vi "Read Logging Interval.vi"(8 "error in (no error)":errorcluster, 11 "Data Logger in":refnum<class "Data Logger.lvclass">) -> (0 "error out":errorcluster, 2 "Logging Interval":dbl=1.0 min=1.0 step=1.0 format="%<%H:%M:%S>t", 3 "Data Logger out":refnum<class "Data Logger.lvclass">)   [LabVIEW 2014, in "Data Logger.lvlib" / "Data Logger.lvclass"]
uses:
  Data Logger.lvclass
  Data Logger.lvclass/Data Logger.ctl
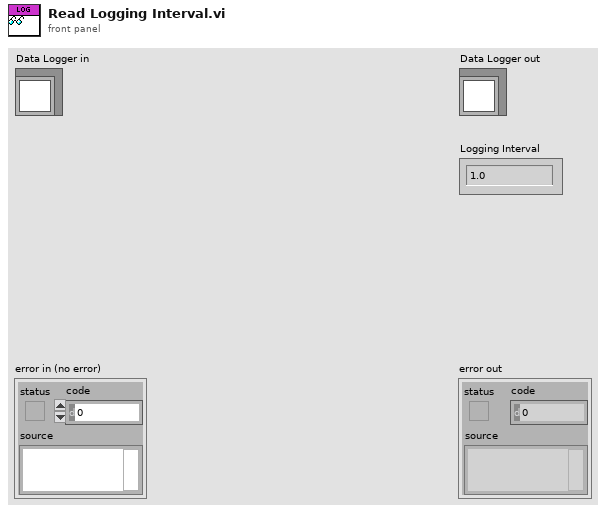
[diagram p1: front panel]
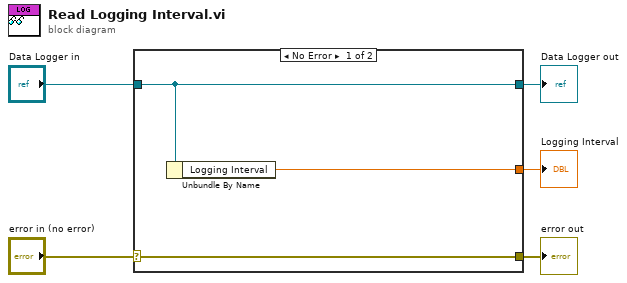
[diagram p0: block diagram]
diagram:
  n1 = case shown="No Error" "error in (no error)" {
    selector: "error in (no error)" -> [w8 w9]
    tunnel: [w8 w9] -> w4
    tunnel: [w7 w10] -> w2
    tunnel: "Data Logger in" -> [w7 w10]
    tunnel: [w6 _] -> w1
    frame No Error {
      n2 = Unbundle By Name(w7) -> ("Logging Interval"=w6:dbl)
    }
    frame Error {
    }
  }
  "error out" <- w4
  "Data Logger out" <- w2
  "Logging Interval" <- w1
